vi "MessageQueue_GetQueue.vi"(1 "Name":string, 3 "OptionalInitValue":T1, 5 "ErrorIn":errorcluster, 9 "CreatIfNotFount (T)":bool=TRUE) -> (14 "QueueOut":refnum<queue>, 17 "CreatedNew":bool, 19 "ErrorOut":errorcluster)   [LabVIEW 2016]
doc: "Erzeugt einen Variant Single Element Queue oder gibt die Referenz zurück, falls der Queue mit diesem Namen bereits existiert\n\nsige / 3.12.13"
uses:
  private/MessageQueue.MessageTypeDef.ctl
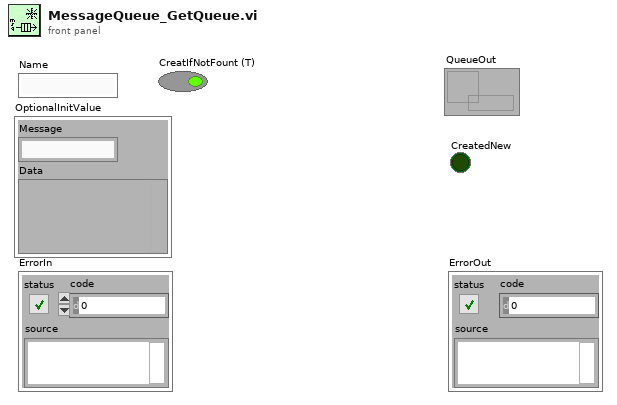
[diagram p1: front panel]
types:
  T1 = typedef "MessageQueue.MessageTypeDef.ctl" = cluster{"Message":string, "Data":variant}
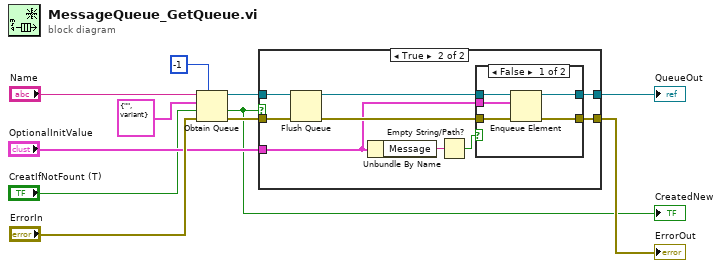
[diagram p0: block diagram]
diagram:
  n1 = Obtain Queue(max queue size (-1, unlimited)=-1, name (unnamed)="Name", element data type=T1 {"Message"="", "Data"=variant} ("Cluster"), create if not found? (T)="CreatIfNotFount (T)", error in (no error)="ErrorIn") -> (queue out=w8:refnum<queue>, created new?=w4:bool, error out=w7:errorcluster)
  "CreatedNew" <- w4
  n2 = case shown="True" w4 {
    tunnel: w8 -> [w13 w22]
    tunnel: w7 -> [w12 w21]
    tunnel: "OptionalInitValue" -> [_ w16]
    tunnel: [w13 w18] -> w2
    tunnel: [w12 w17] -> w5
    frame False {
    }
    frame True {
      n3 = Flush Queue(queue=w22, error in (no error)=w21) -> (queue out=w20:refnum<queue>, error out=w19:errorcluster)  [unwired: 1 out]
      n4 = Unbundle By Name(w16) -> ("Message"=w14:string)
      n5 = Empty String/Path?(string/path=w14) -> (empty?=w15:bool)
      n6 = case shown="False" w15 {
        tunnel: w20 -> [w27 w29]
        tunnel: w19 -> [w26 w28]
        tunnel: [w25 w29] -> w18
        tunnel: [w24 w28] -> w17
        tunnel: w16 -> [w23 _]
        frame False {
          n7 = Enqueue Element(queue=w27, element=w23, error in (no error)=w26) -> (queue out=w25:refnum<queue>, error out=w24:errorcluster)  [unwired: 1 in, 1 out]
        }
        frame True {
        }
      }
    }
  }
  "ErrorOut" <- w5
  "QueueOut" <- w2
